vi "to_json.vi"(8 "error in":errorcluster, 11 "id in":refnum<class "id.lvclass">) -> (0 "error out":errorcluster, 2 "json":string, 3 "id out":refnum<class "id.lvclass">, 4 "Not Default":bool)   [LabVIEW 2020, in "nominal types.lvlib" / "channelFilter.lvlib" / "id.lvclass"]
uses:
  id.lvclass
  id.lvclass/id.ctl
  2098b5ef-f0de-4629-b9a5-4f8fbf79e7eb.vi
  <vilib>/JDP Science/JSONtext/Variant to JSON Text.vi
  <vilib>/JDP Science/JSONtext/LVClass Serializer/JSONtext LVClass Serializer.lvclass
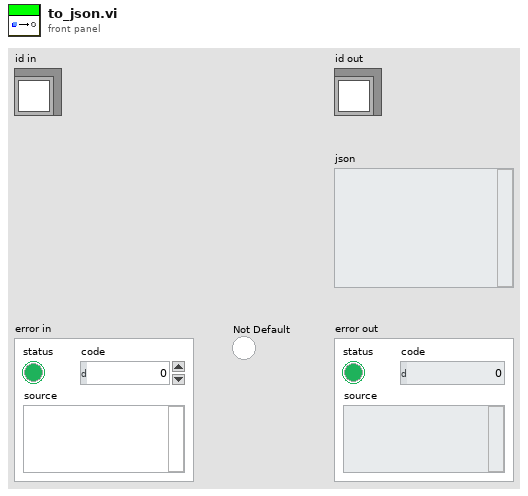
[diagram p1: front panel]
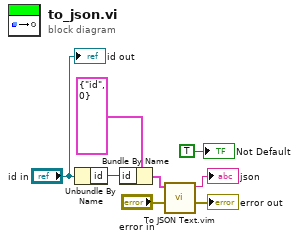
[diagram p0: block diagram]
diagram:
  n1 = Unbundle By Name("id in") -> ("id"=w7:i32)
  n2 = Bundle By Name(cluster=cluster{"type":string, "id":i32} {"type"="id", "id"=0}, "id"=w7) -> (w6:cluster{"type":string, "id":i32})
  n3 = call "To JSON Text.vim"("error in (no error)"="error in", "Anything"=w6) -> ("error out"=→"error out":errorcluster, "<JSON>"=→"json":string)  [unwired: 8 in]
  "id out" <- "id in"
  "Not Default" <- TRUE ("Not Default")
